vi "Read Rank.vi"(8 "error in (no error)":errorcluster, 11 "SG Path Group in":refnum<class "SG 18GHz Path Group.lvclass">) -> (0 "error out":errorcluster, 2 "Rank":dbl, 3 "SG Path Group out":refnum<class "SG 18GHz Path Group.lvclass">)   [LabVIEW 2023, in "RFFixtureCharact.RFPM.lvlib" / "SG 18GHz Path Group.lvclass"]
uses:
  SG 18GHz Path Group.lvclass
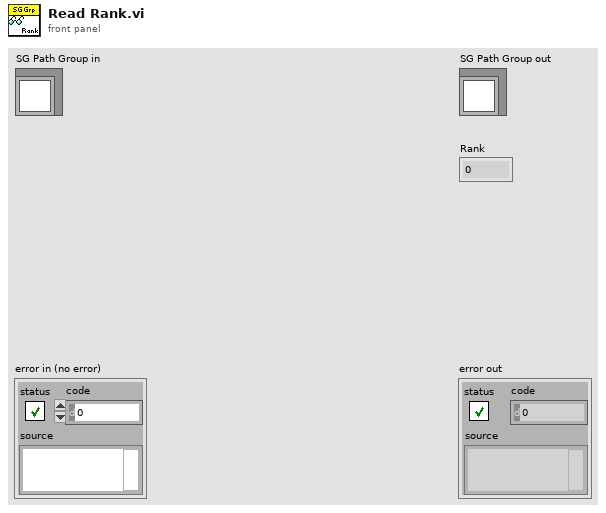
[diagram p1: front panel]
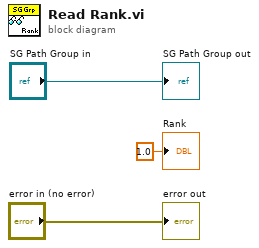
[diagram p0: block diagram]
diagram:
  "error out" <- "error in (no error)"
  "SG Path Group out" <- "SG Path Group in"
  "Rank" <- 1.0 ("Rank")
